vi "UDP Read Memory.vi"(8 "error in (no error)":errorcluster, 9 "超时毫秒(25000)":i32, 11 "UDP Network Connection in":refnum<k16>) -> (0 "error out":errorcluster, 2 "String":string, 3 "UDP Network Connection out":refnum<k16>, 4 "checksum":dbl[](array[numeric]))   [LabVIEW 2017, in "UDP++.lvlib"]
doc: "Reads a split UDP data stream and returns it as a string. The call returns as soon as any bytes arrive and waits the full timeout in ms only when nothing is received."
uses:
  UDP++.lvlib
  a4b2ae4f-aa61-478a-b38d-a9a62d080a2a.vi
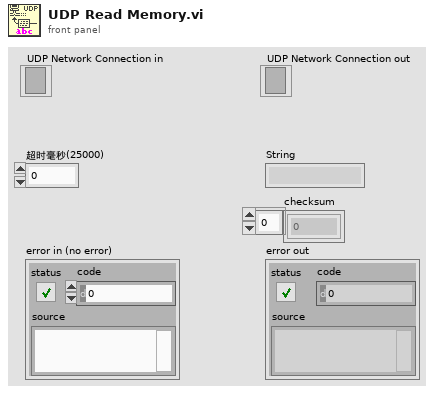
[diagram p1: front panel]
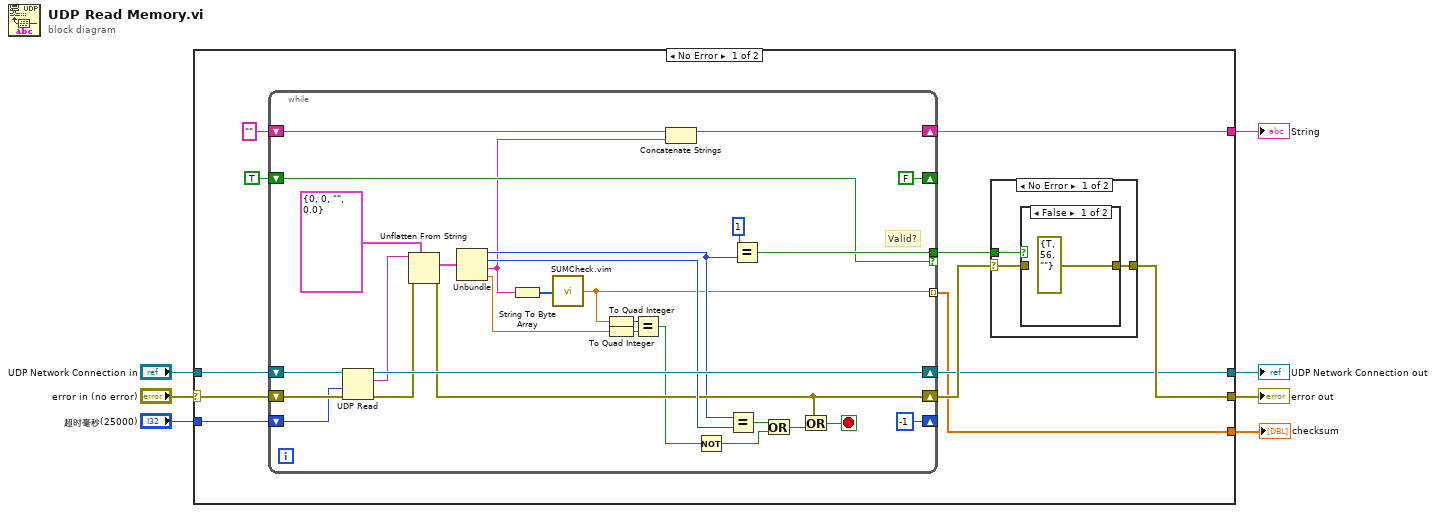
[diagram p0: block diagram]
diagram:
  n1 = case shown="No Error" "error in (no error)" {
    selector: "error in (no error)" -> [w10 w55]
    tunnel: [w18 w55] -> w7
    tunnel: "超时毫秒(25000)" -> [w14 _]
    tunnel: [w13 _] -> w5
    tunnel: [w11 w54] -> w4
    tunnel: "UDP Network Connection in" -> [w9 w54]
    tunnel: [w8 _] -> w1
    frame No Error {
      n2 = while {
        shift-right: [w51] -> w11
        shift-left: w9 -> [w53]
        shift-right: [w40] -> w16
        shift-left: w10 -> [w52]
        shift-right: [w43] -> w13
        shift-left: "" -> [w44]
        shift-right: [-1 ("超时毫秒(25000)")] -> _
        shift-left: w14 -> [w42]
        shift-right: [FALSE] -> _
        shift-left: TRUE -> [w35]
        tunnel: [w36] -> w17 if=w35
        tunnel: [w26] -> w8 mode=indexing
        stop <- w45 stop-if-true
        # "Valid?"
        n3 = UDP Read(connection ID=w53, timeout ms (25000)=w42, 8:w52) -> (data out=w48:string, error out=w47:errorcluster, 3:w51:refnum<k16>)  [unwired: 3 out]
        n4 = Unflatten From String(type=cluster{i32, i32, string, "Validation":dbl} {0, 0, "", "Validation"=0.0} ("output cluster"), binary string=w48, error in (no error)=w47) -> (value=w50:cluster{i32, i32, string, "Validation":dbl}, error out=w40:errorcluster)  [unwired: 2 in, 1 out]
        n5 = Unbundle(w50) -> (w38:i32, w46:i32, w32:string, "Validation"=w29:dbl)
        n6 = String To Byte Array(string=w32) -> (unsigned byte array=w33:u8[])
        n7 = call "SUMCheck.vim"("Array"=w33) -> ("Validation"=w26:dbl)
        n8 = To Quad Integer(1:w26) -> (0:w31:i64)
        n9 = To Quad Integer(1:w29) -> (0:w30:i64)
        n10 = Equal?(x=w31, y=w30) -> (x = y?=w27:bool)
        n11 = Concatenate Strings(w44, w32) -> (w43:string)
        n12 = Not(x=w27) -> (.not. x?=w25:bool)
        n13 = Equal?(x=w38, y=w46) -> (x = y?=w39:bool)
        n14 = Equal?(x=1, y=w38) -> (x = y?=w36:bool)
        n15 = Or(x=w39, y=w25) -> (x .or. y?=w28:bool)
        n16 = Or(x=w40, y=w28) -> (x .or. y?=w45:bool)
      }
      n17 = case shown="No Error" w16 {
        selector: w16 -> [w19 w24]
        tunnel: w17 -> [w21 _]
        tunnel: [w20 w24] -> w18
        frame No Error {
          n18 = case shown="False" w21 {
            tunnel: [errorcluster {"status"=TRUE, "code"=56, "source"=""} ("error IO") w23] -> w20
            tunnel: w19 -> [_ w23]
            frame False {
            }
            frame True {
            }
          }
        }
        frame Error {
        }
      }
    }
    frame Error {
    }
  }
  "error out" <- w7
  "String" <- w5
  "UDP Network Connection out" <- w4
  "checksum" <- w1
